vi "Teleop.vi"(10 "Match Info":T1={"Autonomous Elapsed Seconds"=0.0, "TeleOp Elapsed Seconds"=0.0, "Disabled Elapsed Seconds"=0.0, "Visited Autonomous"=FALSE, "Visited TeleOp"=FALSE, "Visited Disabled"=FALSE, "Autonomous Settings"={"Autonomous Style"=enum."Independent", "VI Refnum"=refnum}}, 11 "Call Context":T2) -> ()   [LabVIEW 2015]
doc: "This VI is called for each enabled TeleOp packet received from the DS. It is typically used to read from joysticks and other inputs and update I/O or setpoints for timed control loops. It should complete and return within 20 milliseconds or risk missing DS packets."
uses:
  <vilib>/Rock Robotics/WPI/DriverStation/WPI_DriverStationDerivedRobotMode.ctl
  <vilib>/Rock Robotics/WPI/DriverStation/WPI_DriverStationMatch Info.ctl
  Drive/Implementation/Global Drive Variables.vi
  <vilib>/Rock Robotics/Network Tables/NT Write Boolean Array.vi
  <vilib>/Rock Robotics/Network Tables/NT Write Numeric Array.vi
  Framework/Robot Global Data.vi
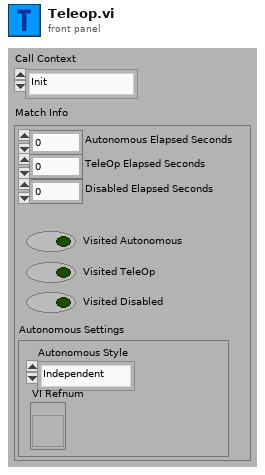
[diagram p1: front panel]
types:
  T1 = typedef "WPI_DriverStationMatch Info.ctl" = cluster{"Autonomous Elapsed Seconds":dbl, "TeleOp Elapsed Seconds":dbl, "Disabled Elapsed Seconds":dbl, "Visited Autonomous":bool, "Visited TeleOp":bool, "Visited Disabled":bool, "Autonomous Settings":cluster{"Autonomous Style":enum16{"Iterative", "Independent"}, "VI Refnum":refnum<vi>}}
  T2 = typedef "WPI_DriverStationDerivedRobotMode.ctl" = enum16{"Init", "Execute", "Stop"}
  T3 = typedef "JoystickData.ctl" = cluster{"Axes":dbl[], "Buttons":bool[]}
  T4 = typedef "Robot Type Def.ctl" = enum32{"Disabled", "Ghost", "Casper", "Lofty", "Board", "RaceRobot", "Casper 2.0", "Excalibot 2.0"}
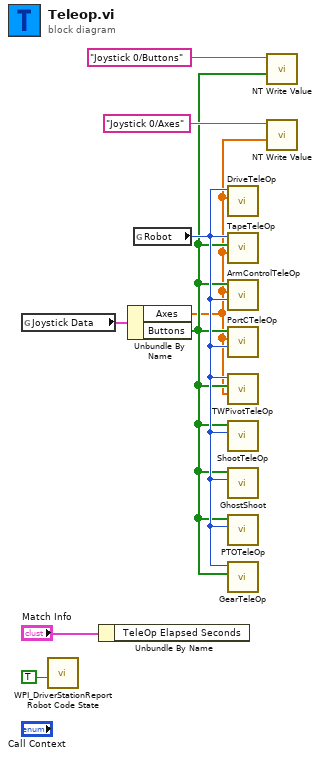
[diagram p0: block diagram]
diagram:
  n1 = global read "Global Drive Variables.vi" "Joystick Data"() -> (w4:T3)
  n2 = call <vilib>:"WPI_DriverStationReport Robot Code State.vi"("TeleOp"=TRUE ("Autonomous")) -> ()  [unwired: 10 in, 1 out]
  n3 = Unbundle By Name("Match Info") -> ()  [unwired: 1 out]
  n4 = Unbundle By Name(w4) -> ("Axes"=w1:dbl[], "Buttons"=w2:bool[])
  n5 = global read "Robot Global Data.vi" "Robot"() -> (w3:T4)
  n6 = call "DriveTeleOp.vi"("Axes"=w1, "Robot"=w3) -> ()  [unwired: 10 in]
  n7 = call "TapeTeleOp.vi"("Axes"=w1, "Buttons"=w2, "Robot"=w3) -> ()  [unwired: 9 in]
  n8 = call "ArmControlTeleOp.vi"("Robot"=w3, "Axes"=w1, "Buttons"=w2) -> ()  [unwired: 9 in]
  n9 = call "PortCTeleOp.vi"("Robot"=w3, "Axes"=w1, "Buttons"=w2) -> ()  [unwired: 9 in]
  n10 = call "TWPivotTeleOp.vi"("Axes"=w1, "Buttons"=w2, "Robot"=w3) -> ()  [unwired: 8 in, 1 out]
  n11 = call "ShootTeleOp.vi"("Robot"=w3, "Buttons"=w2) -> ()  [unwired: 10 in]
  n12 = call "GhostShoot.vi"("Robot"=w3, "Buttons"=w2) -> ()  [unwired: 10 in]
  n13 = call "PTOTeleOp.vi"("Robot"=w3, "Buttons"=w2) -> ()  [unwired: 10 in]
  n14 = call "GearTeleOp.vi"("Buttons"=w2, "Robot"=w3) -> ()  [unwired: 10 in]
  n15 = call-poly <vilib>:"NT Write Value.vi"("Boolean Array"=w2, "Name"="Joystick 0/Buttons") -> ()  [unwired: 9 in, 1 out]
  n16 = call-poly <vilib>:"NT Write Value.vi"("Numeric Array"=w1, "Name"="Joystick 0/Axes") -> ()  [unwired: 9 in, 1 out]
